vi "Check for HW Error.vi"(10 "message in":string, 11 "source in":string) -> (2 "message out":string, 3 "source out":string)   [LabVIEW 2020]
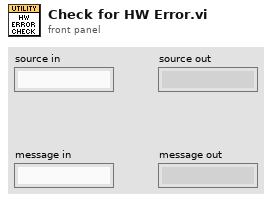
[diagram p1: front panel]
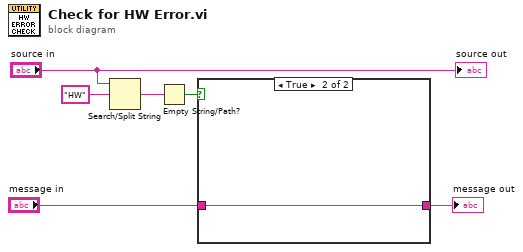
[diagram p0: block diagram]
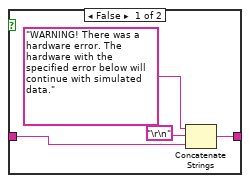
[diagram p2: hidden frame]
diagram:
  n1 = Search/Split String(string="source in", search string/char (-)="HW") -> (match + rest of string=w4:string)  [unwired: 1 in, 2 out]
  n2 = Empty String/Path?(string/path=w4) -> (empty?=w3:bool)
  n3 = case shown="True" w3 {
    tunnel: "message in" -> [w8 w11]
    tunnel: [w10 w11] -> w1
    frame False {
      n4 = Concatenate Strings("WARNING! There was a hardware error. The hardware with the specified error below will continue with simulated data." ("message in"), "\r\n", w8) -> (w10:string)
    }
    frame True {
    }
  }
  "message out" <- w1
  "source out" <- "source in"
